vi "Load CH names into WF-Task list.vi"(8 "error in":errorcluster, 9 "Selected Channels List in":string[](array[string]), 10 "Wfms List":refnum<vi>, 11 "Waveform Task Group refference in":refnum<vi>) -> (0 "error out":errorcluster)   [LabVIEW 2017, in "Waveform-Processing-Custom-Device System Explorer.lvlib"]
doc: "This application uses the reference pointers to update the front panel \"Waveform Group Tasks\" for the channel names in the \"Channel Selection Array\""
uses:
  Waveform-Processing-Custom-Device System Explorer.lvlib
  Types/Channel Selection Array.ctl
  Types/Channel Select items.ctl
  Types/Select Buttons.ctl
panel:
  in  "Channel Selection Array":T1
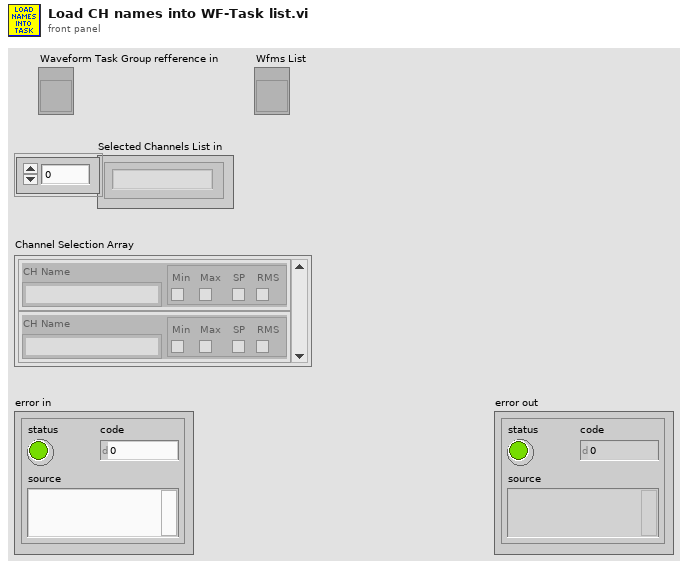
[diagram p1: front panel]
types:
  T1 = typedef "Waveform-Processing-Custom-Device System Explorer.lvlib/Channel Selection Array.ctl" = T2[]
  T2 = typedef "Waveform-Processing-Custom-Device System Explorer.lvlib/Channel Select items.ctl" = cluster{"Buttons":T3, "CH Name":string}
  T3 = typedef "Waveform-Processing-Custom-Device System Explorer.lvlib/Select Buttons.ctl" = cluster{"Min":bool, "Max":bool, "SP":bool, "RMS":bool}
  T4 = typedef "Waveform-Processing-Custom-Device System Explorer.lvlib/Wavefrom Task Group.ctl" = cluster{"Channel Selection Array":T1, "Buttons":T3}
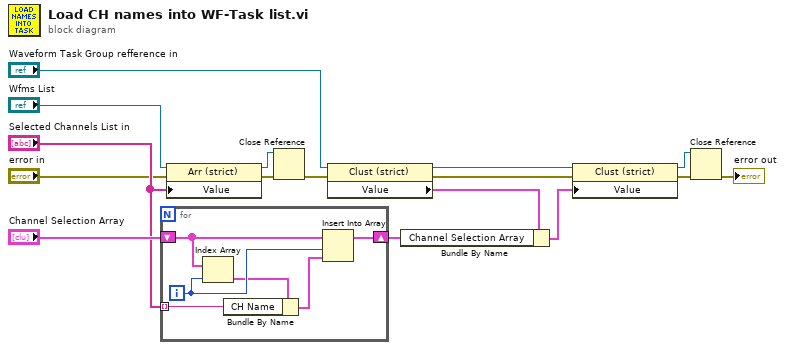
[diagram p0: block diagram]
diagram:
  n1 = for {
    shift-right: [w17] -> w13
    shift-left: "Channel Selection Array" -> [w22]
    tunnel: "Selected Channels List in" -> [w18] mode=indexing
    i -> [w21]
    n2 = Index Array(array=w22, index=w21) -> (element=w20:T2)
    n3 = Bundle By Name(cluster=w20, "CH Name"=w18) -> (w19:T2)
    n4 = Insert Into Array(array=w22, index=w21, new element=w19) -> (w17:T1)
  }
  n5 = property class="Arr (strict)"(reference="Wfms List", error in="error in", "Value"="Selected Channels List in") -> (reference out=w8:refnum<vi>, error out=w7:errorcluster)
  n6 = Close Reference(reference=w8, error in (no error)=w7) -> (error out=w4:errorcluster)
  n7 = property class="Clust (strict)"(reference="Waveform Task Group refference in", error in=w4) -> (reference out=w10:refnum<vi>, error out=w15:errorcluster, "Value"=w12:T4)
  n8 = Bundle By Name(cluster=w12, "Channel Selection Array"=w13) -> (w5:T4)
  n9 = property class="Clust (strict)"(reference=w10, error in=w15, "Value"=w5) -> (reference out=w9:refnum<vi>, error out=w11:errorcluster)
  n10 = Close Reference(reference=w9, error in (no error)=w11) -> (error out=→"error out":errorcluster)
